vi "manual_test_wait.vi"(5 "change_in_event":refnum<user-event>, 7 "waitgroup":T1, 8 "error in (no error)":errorcluster, 11 "data":variant) -> (0 "error out":errorcluster)   [LabVIEW 2015, in "example_01.lvlib"]
uses:
  example_01.lvlib
  <userlib>/antonio-alexander/lv-waitgroup/public/_controls/api_waitgroup.ctl
  lv-recipe-machine/public/_controls/change.ctl
  _controls/step_data.ctl
  _controls/manual_actions.ctl
  lv-recipe-machine/lv-recipe-machine.lvlib
  <userlib>/antonio-alexander/lv-waitgroup/lv-waitgroup.lvlib
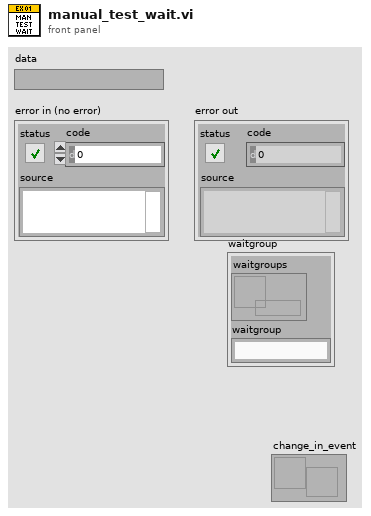
[diagram p1: front panel]
types:
  T1 = typedef "lv-waitgroup.lvlib/api_waitgroup.ctl" = cluster{"waitgroups":refnum<data-value>, "waitgroup":string}
  T2 = typedef "example_01.lvlib/manual_actions.ctl" = enum16{"<manual_action>", "manual_test_random", "manual_test_comparison", "manual_test_wait", "<null>"}
  T3 = typedef "example_01.lvlib/step_data.ctl" = cluster{"data":variant, "step":string}
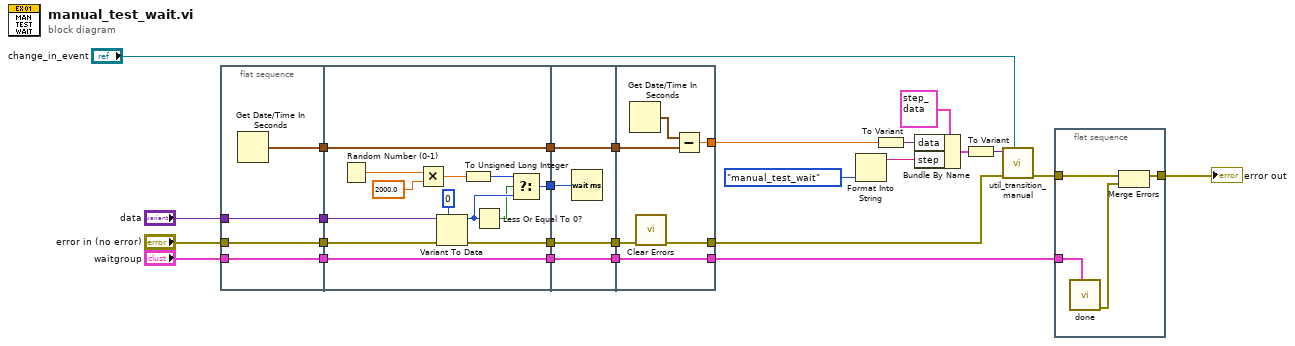
[diagram p0: block diagram]
diagram:
  n1 = flat-sequence {
    tunnel: "data" -> [w30]
    tunnel: "error in (no error)" -> [w29]
    tunnel: [w30] -> w21
    tunnel: [w29] -> w20
    tunnel: [w28] -> w19
    tunnel: "waitgroup" -> [w27]
    tunnel: [w27] -> w5
    tunnel: w21 -> [w36]
    tunnel: w20 -> [w37]
    tunnel: w19 -> [w43]
    tunnel: [w43] -> w18
    tunnel: [w35] -> w16
    tunnel: [w32] -> w10
    tunnel: w5 -> [w31]
    tunnel: [w31] -> w4
    tunnel: w18 -> [w47]
    tunnel: [w47] -> w17
    tunnel: w16 -> [w46]
    tunnel: [w45] -> w11
    tunnel: w10 -> [w45]
    tunnel: w4 -> [w44]
    tunnel: [w44] -> w3
    tunnel: w17 -> [w52]
    tunnel: [w51] -> w15
    tunnel: [w50] -> w12
    tunnel: w11 -> [w49]
    tunnel: w3 -> [w48]
    tunnel: [w48] -> w2
    frame #0 {
      n2 = Get Date/Time In Seconds() -> (seconds since 1Jan1904=w28:timestamp)
    }
    frame #1 {
      n3 = Random Number (0-1)() -> (number: 0 to 1=w39:dbl)
      n4 = Multiply(x=w39, y=2000.0) -> (x*y=w41:dbl)
      n5 = Variant To Data(error in=w37, type=u32 0, Variant=w36) -> (data=w34:u32, error out=w32:errorcluster)
      n6 = To Unsigned Long Integer(number=w41) -> (unsigned 32bit integer=w42:u32)
      n7 = Less Or Equal To 0?(x=w34) -> (x <= 0?=w33:bool)
      n8 = Select(t=w42, s=w33, f=w34) -> (s? t:f=w35:u32)
    }
    frame #2 {
      n9 = Wait (ms)(milliseconds to wait=w46) -> ()  [unwired: 1 out]
    }
    frame #3 {
      n10 = Get Date/Time In Seconds() -> (seconds since 1Jan1904=w53:timestamp)
      n11 = call <vilib>:"Clear Errors.vi"("error in (no error)"=w49) -> ("error out"=w50:errorcluster)  [unwired: 5 in, 1 out]
      n12 = Subtract(x=w53, y=w52) -> (x-y=w51:dbl)
    }
  }
  n13 = Format Into String(manual_actions."manual_test_wait" ("manual_action")) -> (resulting string=w25:string)  [unwired: 3 in, 1 out]
  n14 = To Variant(anything=w15) -> (Variant=w24:variant)
  n15 = Bundle By Name(cluster=T3 {"data"=variant, "step"=""}, "data"=w24, "step"=w25) -> (w13:T3)
  n16 = To Variant(anything=w13) -> (Variant=w9:variant)
  n17 = call "util_transition_manual.vi"("change_in_event"="change_in_event", "error in (no error)"=w12, "data"=w9) -> ("error out"=w7:errorcluster)  [unwired: 8 in]
  n18 = flat-sequence {
    tunnel: w7 -> [w57]
    tunnel: [w56] -> w1
    tunnel: w2 -> [w54]
    frame #0 {
      n19 = call <userlib>:"done.vi"("waitgroup"=w54) -> ("error out"=w55:errorcluster)  [unwired: 10 in]
      n20 = Merge Errors(w57, w55) -> (w56:errorcluster)
    }
  }
  "error out" <- w1
